vi "Control Pnuematics.vi"(11 "Loop Time (ms)":u32) -> ()   [LabVIEW 2017]
uses:
  <vilib>/Rock Robotics/WPI/Utilities/WPI_GetSetVariantRefNum.vi
  Globals/Robot Global Data.vi
  <vilib>/Rock Robotics/WPI/Solenoid/WPI_SolenoidSetEnum.vi
  <vilib>/Rock Robotics/WPI/Solenoid/Deprecated/WPI_SolenoidSetBool.vi
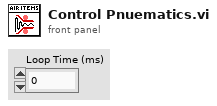
[diagram p1: front panel]
types:
  T1 = typedef "WPI_SolenoidDevRef.ctl" = cluster{"DevStatus":errorcluster, "Pneumatics Control Module":u8, "Forward Solenoid Channel":T2, "Reverse Solenoid Channel":T2}
  T2 = typedef "WPI_SolenoidChannel.ctl" = enum8{"Solenoid 0", "Solenoid 1", "Solenoid 2", "Solenoid 3", "Solenoid 4", "Solenoid 5", "Solenoid 6", "Solenoid 7", "Invalid"}
  T3 = typedef "WPI_CompressorDevRef.ctl" = cluster{"DevStatus":errorcluster, "Pneumatics Control Module":u8}
  T4 = typedef "WPI_SolenoidValue.ctl" = enum16{"Off", "On", "Forward", "Reverse"}
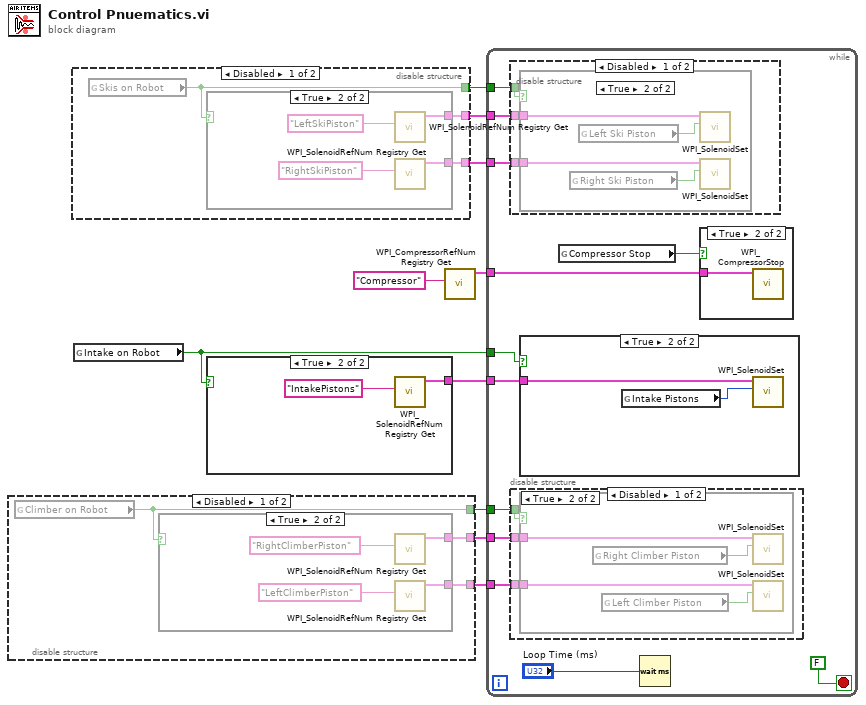
[diagram p0: block diagram]
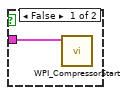
[diagram p12: hidden frame]
diagram:
  n1 = disable-structure shown="Disabled" {
    disable-tunnel: [w13 _] -> w5
    disable-tunnel: [w12 _] -> w4
    disable-tunnel: [w11 _] -> w1
    frame Disabled {
      n2 = global read "Robot Global Data.vi" "Climber on Robot"() -> (w11:bool)
      n3 = case shown="True" w11 {
        tunnel: [_ w17] -> w13
        tunnel: [_ w14] -> w12
        frame False {
        }
        frame True {
          n4 = call <vilib>:"WPI_SolenoidRefNum Registry Get.vi"("refnum name"="RightClimberPiston") -> ("SolenoidDevRef"=w17:T1)  [unwired: 9 in, 1 out]
          n5 = call <vilib>:"WPI_SolenoidRefNum Registry Get.vi"("refnum name"="LeftClimberPiston") -> ("SolenoidDevRef"=w14:T1)  [unwired: 9 in, 1 out]
        }
      }
    }
    frame Enabled {
    }
  }
  n6 = disable-structure shown="Disabled" {
    disable-tunnel: [w20 _] -> w7
    disable-tunnel: [w19 _] -> w6
    disable-tunnel: [w18 _] -> w2
    frame Disabled {
      n7 = global read "Robot Global Data.vi" "Skis on Robot"() -> (w18:bool)
      n8 = case shown="True" w18 {
        tunnel: [_ w24] -> w20
        tunnel: [_ w21] -> w19
        frame False {
        }
        frame True {
          n9 = call <vilib>:"WPI_SolenoidRefNum Registry Get.vi"("refnum name"="LeftSkiPiston") -> ("SolenoidDevRef"=w24:T1)  [unwired: 9 in, 1 out]
          n10 = call <vilib>:"WPI_SolenoidRefNum Registry Get.vi"("refnum name"="RightSkiPiston") -> ("SolenoidDevRef"=w21:T1)  [unwired: 9 in, 1 out]
        }
      }
    }
    frame Enabled {
    }
  }
  n11 = global read "Robot Global Data.vi" "Intake on Robot"() -> (w3:bool)
  n12 = case shown="True" w3 {
    tunnel: [_ w26] -> w8
    frame False {
    }
    frame True {
      n13 = call <vilib>:"WPI_SolenoidRefNum Registry Get.vi"("refnum name"="IntakePistons") -> ("SolenoidDevRef"=w26:T1)  [unwired: 9 in, 1 out]
    }
  }
  n14 = call <vilib>:"WPI_CompressorRefNum Registry Get.vi"("refnum name"="Compressor") -> ("CompressorDevRef"=w9:T3)  [unwired: 9 in, 1 out]
  n15 = while {
    tunnel: w9 -> [w37]
    tunnel: w8 -> [w34]
    tunnel: w7 -> [w33]
    tunnel: w6 -> [w32]
    tunnel: w4 -> [w30]
    tunnel: w5 -> [w31]
    tunnel: w3 -> [w29]
    tunnel: w2 -> [w28]
    tunnel: w1 -> [w27]
    stop <- FALSE stop-if-true
    n16 = disable-structure shown="Disabled" {
      disable-tunnel: w33 -> [w48 _]
      disable-tunnel: w32 -> [w47 _]
      disable-tunnel: w28 -> [w46 _]
      frame Disabled {
        n17 = case shown="True" w46 {
          tunnel: w48 -> [_ w52]
          tunnel: w47 -> [_ w49]
          frame False {
          }
          frame True {
            n18 = global read "Robot Global Data.vi" "Right Ski Piston"() -> (w50:bool)
            n19 = global read "Robot Global Data.vi" "Left Ski Piston"() -> (w51:bool)
            n20 = call-poly <vilib>:"WPI_SolenoidSet.vi"("Value"=w51, "SolenoidDevRef"=w52) -> ()  [unwired: 8 in, 2 out]
            n21 = call-poly <vilib>:"WPI_SolenoidSet.vi"("Value"=w50, "SolenoidDevRef"=w49) -> ()  [unwired: 8 in, 2 out]
          }
        }
      }
      frame Enabled {
      }
    }
    n22 = disable-structure shown="Disabled" {
      disable-tunnel: w31 -> [w41 _]
      disable-tunnel: w30 -> [w40 _]
      disable-tunnel: w27 -> [w39 _]
      frame Disabled {
        n23 = case shown="True" w39 {
          tunnel: w41 -> [_ w45]
          tunnel: w40 -> [_ w42]
          frame False {
          }
          frame True {
            n24 = global read "Robot Global Data.vi" "Right Climber Piston"() -> (w44:bool)
            n25 = global read "Robot Global Data.vi" "Left Climber Piston"() -> (w43:bool)
            n26 = call-poly <vilib>:"WPI_SolenoidSet.vi"("Value"=w44, "SolenoidDevRef"=w45) -> ()  [unwired: 8 in, 2 out]
            n27 = call-poly <vilib>:"WPI_SolenoidSet.vi"("Value"=w43, "SolenoidDevRef"=w42) -> ()  [unwired: 8 in, 2 out]
          }
        }
      }
      frame Enabled {
      }
    }
    n28 = case shown="True" w29 {
      tunnel: w34 -> [_ w54]
      frame False {
      }
      frame True {
        n29 = global read "Robot Global Data.vi" "Intake Pistons"() -> (w53:T4)
        n30 = call-poly <vilib>:"WPI_SolenoidSet.vi"("Value"=w53, "SolenoidDevRef"=w54) -> ()  [unwired: 8 in, 2 out]
      }
    }
    n31 = global read "Robot Global Data.vi" "Compressor Stop"() -> (w38:bool)
    n32 = Wait (ms)(milliseconds to wait="Loop Time (ms)") -> ()  [unwired: 1 out]
    n33 = case shown="True" w38 {
      tunnel: w37 -> [w55 w56]
      frame False {
        n34 = call <vilib>:"WPI_CompressorStart.vi"("CompressorDevRef"=w55) -> ()  [unwired: 9 in, 2 out]
      }
      frame True {
        n35 = call <vilib>:"WPI_CompressorStop.vi"("CompressorDevRef"=w56) -> ()  [unwired: 9 in, 2 out]
      }
    }
  }
